vi "Process Outgoing Frames.vi"(8 "error in (no error)":errorcluster, 9 "timeout ms":i32=100, 11 "Variables":T1={"Process Ref"=refnum, "Comm Ref"=refnum, "Data Refs"={"ProtectionsAndCounters.Ref"=refnum, "Signals.Ref"=refnum, "Status.Ref"=refnum, "Overrides"=refnum, "IncomingSignals.Ref"=refnum, "CtrandProtctnVld.Ref"=refnum, "RcvTime.Ref"=refnum, "TimeDiff.Ref"=refnum, "IncomingProtCtr.Ref"=refnum}, "Settings"={"Name"="", "Priority"=0, "XNET Settings"={"Database"="", "Cluster"="", "Port"="", "Baud rate [Bd]"=0, "Termination"=0, "CAN I/O Mode"=0, "FD Baud rate [Bd]"=500000, "Priority"=100, "Use Legacy"=FALSE, "FD ISO Mode"=0}, "FPGA Session"=0, "Outgoing CAN Session"="", "Outgoing Frame Count"=0, "Outgoing Frames"=[], "Incoming CAN Session"="", "Incoming Frame Count"=0, "Incoming Frames"=[], "Incoming Values"={"Signal Values"=[], "Signal Invalid Values"=[], "ProtCtr Sig Values"=[], "Timestamps"=[], "Time Differences"=[], "IDs"=[]}}, "Stream Refs"={"Addon"="", "Port"="", "Filter Ref"=refnum, "Default Filter"={"ID Filters"=[], "Direction Filter"=enum."Tx/Rx", "Type Filter"=enum."All"}, "Port Settings"={"Mode"=0, "Baud Rate"=0, "Termination"=0, "FD ISO Mode"=0, "FD Baud Rate"=0}}} {"Stream Refs"."Port Settings"."FD ISO Mode" items=["ISO", "Non ISO", "ISO Legacy"]; "Stream Refs"."Port Settings"."Termination" items=["Off", "On"]; "Stream Refs"."Port Settings"."Mode" items=["CAN 2.0", "CAN FD", "CAN FD+BRS"]; "Settings"."XNET Settings"."FD ISO Mode" items=["ISO", "Non ISO", "ISO Legacy"]; "Settings"."XNET Settings"."CAN I/O Mode" items=["CAN 2.0", "CAN FD", "CAN FD+BRS"]; "Settings"."XNET Settings"."Termination" items=["Off", "On"]}) -> (0 "error out":errorcluster, 3 "Variables out":T1={"Process Ref"=refnum, "Comm Ref"=refnum, "Data Refs"={"ProtectionsAndCounters.Ref"=refnum, "Signals.Ref"=refnum, "Status.Ref"=refnum, "Overrides"=refnum, "IncomingSignals.Ref"=refnum, "CtrandProtctnVld.Ref"=refnum, "RcvTime.Ref"=refnum, "TimeDiff.Ref"=refnum, "IncomingProtCtr.Ref"=refnum}, "Settings"={"Name"="", "Priority"=0, "XNET Settings"={"Database"="", "Cluster"="", "Port"="", "Baud rate [Bd]"=0, "Termination"=0, "CAN I/O Mode"=0, "FD Baud rate [Bd]"=500000, "Priority"=100, "Use Legacy"=FALSE, "FD ISO Mode"=0}, "FPGA Session"=0, "Outgoing CAN Session"="", "Outgoing Frame Count"=0, "Outgoing Frames"=[], "Incoming CAN Session"="", "Incoming Frame Count"=0, "Incoming Frames"=[], "Incoming Values"={"Signal Values"=[], "Signal Invalid Values"=[], "ProtCtr Sig Values"=[], "Timestamps"=[], "Time Differences"=[], "IDs"=[]}}, "Stream Refs"={"Addon"="", "Port"="", "Filter Ref"=refnum, "Default Filter"={"ID Filters"=[], "Direction Filter"=enum."Tx/Rx", "Type Filter"=enum."All"}, "Port Settings"={"Mode"=0, "Baud Rate"=0, "Termination"=0, "FD ISO Mode"=0, "FD Baud Rate"=0}}} {"Stream Refs"."Port Settings"."FD ISO Mode" items=["ISO", "Non ISO", "ISO Legacy"]; "Stream Refs"."Port Settings"."Termination" items=["Off", "On"]; "Stream Refs"."Port Settings"."Mode" items=["CAN 2.0", "CAN FD", "CAN FD+BRS"]; "Settings"."XNET Settings"."FD ISO Mode" items=["ISO", "Non ISO", "ISO Legacy"]; "Settings"."XNET Settings"."CAN I/O Mode" items=["CAN 2.0", "CAN FD", "CAN FD+BRS"]; "Settings"."XNET Settings"."Termination" items=["Off", "On"]})   [LabVIEW 2019, in "Ghost Bus Addon Engine.lvlib"]
uses:
  Ghost Bus Addon Engine.lvlib
  Types/RT Async Engine Variables.ctl
  <vilib>/NI/NIVS Inline Async API/_VS Inline Async API/Process/Process.lvclass
  <vilib>/NI/NI VeriStand Addon Network Comm/Engine/VeriStand Comm.lvclass
  Types/RT Data References.ctl
  <vilib>/NI/NIVS Inline Async API/_Data Access Engine/Data Access Engine/Types/Write.DVR.ctl
  <vilib>/NI/NIVS Inline Async API/_Data Access Engine/Access Type Classes/Write/Write.lvclass
  <vilib>/NI/NIVS Inline Async API/_Data Access Engine/Data Access Engine/Types/Read.DVR.ctl
  <vilib>/NI/NIVS Inline Async API/_Data Access Engine/Access Type Classes/Read/Read.lvclass
  Types/RT Async Engine Settings.ctl
  Addon Shared/Types/XNET Settings.ctl
  SubModules/Frame-Protection-Support/Source/Engine/Types/RT Frame Settings.ctl
  SubModules/Frame-Protection-Support/Source/Shared/Types/Exported Frame Type.ctl
  SubModules/Frame-Protection-Support/Source/Engine/Types/RT Protection Configuration.ctl
  SubModules/Frame-Protection-Support/Source/Shared/Types/Protection Type.ctl
  SubModules/Frame-Protection-Support/Source/Shared/Types/XNET Signal Configuration.ctl
  SubModules/Frame-Protection-Support/Source/Shared/Types/Exported Counter Settings.ctl
  SubModules/Frame-Protection-Support/Source/Shared/Types/Exported Event Trigger Type.ctl
  SubModules/Frame-Protection-Support/Source/Engine/Types/RT Frame Incoming Values.ctl
  SubModules/CAN-Streaming-Support/Source/Addon/Addon Engine/Types/Engine Stream Refs.ctl
  SubModules/CAN-Streaming-Support/Source/Addon/Addon Shared/Types/Direction Filter.ctl
  SubModules/CAN-Streaming-Support/Source/Addon/Addon Shared/Types/Type Filter.ctl
  SubModules/CAN-Streaming-Support/Source/Addon/Addon Shared/Types/Filter Parameters.ctl
  SubModules/CAN-Streaming-Support/Source/Addon/Addon Engine/Types/Engine Stream Port Settings.ctl
  <vilib>/NI/NIVS Inline Async API/_Data Access Engine/Access Type Classes/Read/Read.lvclass/Read.ctl
  <vilib>/NI/NIVS Inline Async API/_Data Access Engine/Access Type Classes/Write/Write.lvclass/Write.ctl
  <vilib>/NI/NIVS Inline Async API/_Data Access Engine/Data Access Engine/Methods/Write.Data.vi
  <vilib>/NI/NIVS Inline Async API/_Data Access Engine/Access Type Classes/Write/Write.ProcessData.vi
  <vilib>/NI/NIVS Inline Async API/_Data Access Engine/Data Access Engine/Methods/Read.Data.Detect.vi
  <vilib>/NI/NIVS Inline Async API/_Data Access Engine/Data Access Engine/Methods/Read.Data.vi
  SubModules/Frame-Protection-Support/Source/Engine/SubVIs/Determine Transmit.vi
  SubModules/Frame-Protection-Support/Source/Engine/SubVIs/Update Counter Signals.vi
  SubModules/Frame-Protection-Support/Source/Engine/SubVIs/Get Frame Data.vi
  SubModules/Frame-Protection-Support/Source/Engine/SubVIs/Convert EU Data to XNET Frame.vi
  SubModules/Frame-Protection-Support/Source/Engine/SubVIs/Update Protection Signals.vi
  SubModules/Frame-Protection-Support/Source/Engine/SubVIs/Determine Disabled.vi
  <vilib>/NI/NIVS Inline Async API/_Data Access Engine/Data Access Engine/Methods/Write.Data.Commit.vi
  <vilib>/NI/NIVS Inline Async API/_Data Access Engine/Access Type Classes/Write/Write.Buffer.vi
  <vilib>/NI/NIVS Inline Async API/_Data Access Engine/Access Type Classes/Write/Write.Commit.vi
  <vilib>/NI/NIVS Inline Async API/_Data Access Engine/Access Type Classes/Read/Read.ProcessData.Detect.vi
  <vilib>/NI/NIVS Inline Async API/_Data Access Engine/Access Type Classes/Read/Read.ProcessData.vi
  SubModules/Frame-Protection-Support/Source/Engine/SubVIs/Determine Transmission.vi
  SubModules/Frame-Protection-Support/Source/Engine/SubVIs/Determine Periodic.vi
  SubModules/Frame-Protection-Support/Source/Engine/SubVIs/Set Counter Signal.vi
  SubModules/Frame-Protection-Support/Source/Engine/SubVIs/Calculate Counter Value.vi
  SubModules/Frame-Protection-Support/Source/Engine/SubVIs/Set Protection Signal.vi
  SubModules/Frame-Protection-Support/Source/Engine/SubVIs/Calculate Protection Value.vi
  <vilib>/NI/NIVS Inline Async API/_Data Access Engine/Data Access Engine/Methods/Write.Data.Buffer.vi
  SubModules/Frame-Protection-Support/Source/Engine/SubVIs/Get Protection Signals.vi
  <vilib>/xnet/xnet.llb/XNET Convert.vi
  <vilib>/xnet/xnet.llb/XNET Convert (Signal to Frame Raw).vi
  <vilib>/xnet/xnet.llb/XNET Convert (Signal to Frame CAN).vi
  <vilib>/xnet/xnet.llb/XNET Write (Frame CAN).vi
  <vilib>/NI/NIVS Inline Async API/_Data Access Engine/Data Access Engine/Data Access Engine.lvclass
  SubModules/Frame-Protection-Support/Source/Engine/Protection and Counter Support Engine.lvlib
  SubModules/Frame-Protection-Support/Source/Shared/Protection and Counter Support Shared.lvlib
  SubModules/CAN-Streaming-Support/Source/Addon/Addon Shared/CAN Stream Support Shared.lvlib
  SubModules/CAN-Streaming-Support/Source/Addon/Addon Engine/CAN Stream Support Engine.lvlib
  Addon Shared/Ghost Bus Addon Shared.lvlib
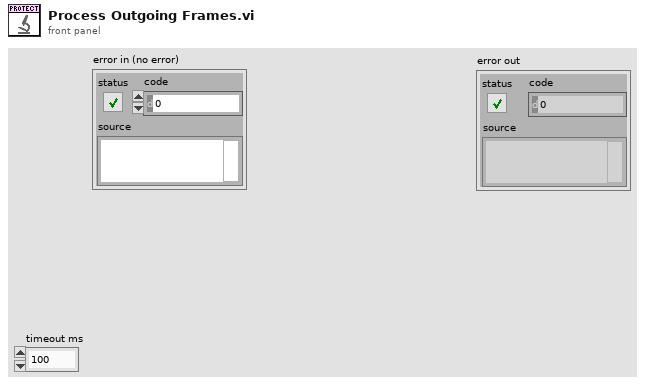
[diagram p1: front panel]
types:
  T1 = typedef "Ghost Bus Addon Engine.lvlib/RT Async Engine Variables.ctl" = cluster{"Process Ref":refnum<class "Process.lvclass">, "Comm Ref":refnum<class "VeriStand Comm.lvclass">, "Data Refs":T2, "Settings":T5, "Stream Refs":T15}
  T2 = typedef "Ghost Bus Addon Engine.lvlib/RT Data References.ctl" = cluster{"ProtectionsAndCounters.Ref":T3, "Signals.Ref":T4, "Status.Ref":T3, "Overrides":T4, "IncomingSignals.Ref":T3, "CtrandProtctnVld.Ref":T3, "RcvTime.Ref":T3, "TimeDiff.Ref":T3, "IncomingProtCtr.Ref":T3}
  T3 = typedef "Data Access Engine.lvlib/Data Access Engine.lvclass/Write.DVR.ctl" = refnum<data-value>
  T4 = typedef "Data Access Engine.lvlib/Data Access Engine.lvclass/Read.DVR.ctl" = refnum<data-value>
  T5 = typedef "Ghost Bus Addon Engine.lvlib/RT Async Engine Settings.ctl" = cluster{"Name":string, "Priority":i32, "XNET Settings":T6, "FPGA Session":u32, "Outgoing CAN Session":refnum<k21>, "Outgoing Frame Count":i32, "Outgoing Frames":T7[], "Incoming CAN Session":refnum<k21>, "Incoming Frame Count":i32, "Incoming Frames":T7[], "Incoming Values":T14}
  T6 = typedef "Ghost Bus Addon Shared.lvlib/XNET Settings.ctl" = cluster{"Database":refnum<k21>, "Cluster":refnum<k21>, "Port":string, "Baud rate [Bd]":u64, "Termination":u32, "CAN I/O Mode":u32, "FD Baud rate [Bd]":u64, "Priority":i32, "Use Legacy":bool, "FD ISO Mode":u32}
  T7 = typedef "Protection and Counter Support Engine.lvlib/RT Frame Settings.ctl" = cluster{"Type":T8, "Frame ID":u32, "Payload Length":u32, "VS Offset":i32, "VS Length":i32, "Frame Conversion":refnum<k21>, "Frame.Data":dbl[], "Generation Period":u32, "Time Since Last Generation":u32, "Generation Iterations":u32, "Generation Counter":u32, "Has Protection?":bool, "Protection Configurations":T9[], "Has Counter?":bool, "Counter Configurations":T12[], "Has Disable?":bool, "Disable VS Index":i32, "Transmit Trigger":T13, "Trigger VS Index":i32}
  T8 = typedef "Protection and Counter Support Shared.lvlib/Exported Frame Type.ctl" = enum16{"Periodic", "Event", "Periodic/Event"}
  T9 = typedef "Protection and Counter Support Engine.lvlib/RT Protection Configuration.ctl" = cluster{"Protection Frame Index":i32, "Protection Type":T10, "Data Indeces":i32[], "Data Array":dbl[], "Check Sum Conversion":refnum<k21>, "CRC Channels":T11[], "Protection VS Index":i32, "Counter Data Index":i32, "Override Index":i32, "Override Value Index":i32}
  T10 = typedef "Protection and Counter Support Shared.lvlib/Protection Type.ctl" = enum16{"Arb ID + Bytes Checksum with Inversion", "Arb ID + Bytes CRC with Inversion", "Reversed Raw Signal Checksum with Inversion", "Concatenated Two's Compliment"}
  T11 = typedef "Protection and Counter Support Shared.lvlib/XNET Signal Configuration.ctl" = cluster{"Start Bit":i32, "Name":string, "Number of bits":i32, "Scale":dbl, "Offset":dbl, "Data Type":u32, "Counter":bool}
  T12 = typedef "Protection and Counter Support Shared.lvlib/Exported Counter Settings.ctl" = cluster{"Frame Index":i32, "Max Count":dbl, "VS Index":i32, "Bit Length":i64, "Override Index":i32, "Override Value Index":i32}
  T13 = typedef "Protection and Counter Support Shared.lvlib/Exported Event Trigger Type.ctl" = enum16{"Channel value change", "Trigger channel (not zero)", "Channel value change or trigger channel (not zero)", "Trigger channel (any value change)", "Channel value change or trigger channel (any value change)"}
  T14 = typedef "Protection and Counter Support Engine.lvlib/RT Frame Incoming Values.ctl" = cluster{"Signal Values":dbl[], "Signal Invalid Values":dbl[], "ProtCtr Sig Values":dbl[], "Timestamps":timestamp[], "Time Differences":dbl[], "IDs":u32[]}
  T15 = typedef "CAN Stream Support Engine.lvlib/Engine Stream Refs.ctl" = cluster{"Addon":string, "Port":refnum<k21>, "Filter Ref":refnum<data-value>, "Default Filter":T16, "Port Settings":T19}
  T16 = typedef "CAN Stream Support Shared.lvlib/Filter Parameters.ctl" = cluster{"ID Filters":u32[], "Direction Filter":T17, "Type Filter":T18}
  T17 = typedef "CAN Stream Support Shared.lvlib/Direction Filter.ctl" = enum16{"Tx/Rx", "Rx", "Tx"}
  T18 = typedef "CAN Stream Support Shared.lvlib/Type Filter.ctl" = enum16{"All", "CAN Data", "CAN Remote", "CAN Bus Error", "CAN 2.0 Data", "CAN FD Data", "CAN FD+BRS Data", "J1939 Data", "Delay", "Log Trigger", "Start Trigger"}
  T19 = typedef "CAN Stream Support Engine.lvlib/Engine Stream Port Settings.ctl" = cluster{"Mode":u32, "Baud Rate":u64, "Termination":u32, "FD ISO Mode":u32, "FD Baud Rate":u64}
  T20 = typedef "XNET Frame CAN.ctl" = cluster{"timestamp":timestamp, "payload":u8[], "identifier":u32, "type":T21, "extended?":bool, "echo?":bool}
  T21 = typedef "XNET Frame Type CAN.ctl" = u8
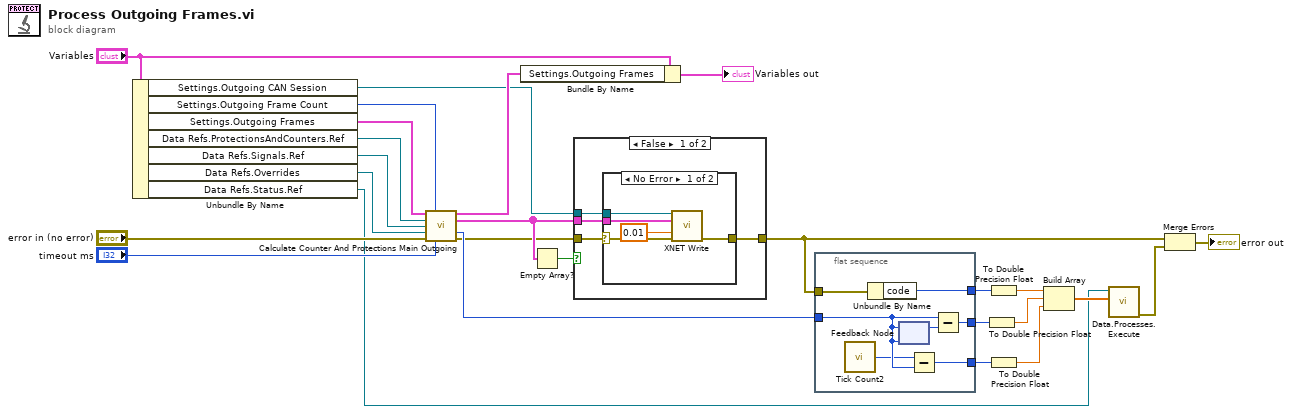
[diagram p0: block diagram]
diagram:
  n1 = Unbundle By Name("Variables") -> ("Settings.Outgoing CAN Session"=w10:refnum<k21>, "Settings.Outgoing Frame Count"=w24:i32, "Settings.Outgoing Frames"=w7:T7[], "Data Refs.ProtectionsAndCounters.Ref"=w2:T3, "Data Refs.Signals.Ref"=w3:T4, "Data Refs.Overrides"=w1:T4, "Data Refs.Status.Ref"=w4:T3)
  n2 = call "Calculate Counter And Protections Main Outgoing.vi"("Frames in"=w7, "Frame Count"=w24, "Protections"=w2, "Signals"=w3, "Overrides"=w1, "error in (no error)"="error in (no error)", "timeout ms"="timeout ms") -> ("Frames out"=w14:T7[], "Frames"=w13:T20[], "Tick Count(uSec)"=w22:u32, "error out"=w9:errorcluster)  [unwired: 5 in]
  n3 = Bundle By Name(cluster="Variables", "Settings.Outgoing Frames"=w14) -> (→"Variables out":T1)
  n4 = Empty Array?(array=w13) -> (empty?=w12:bool)
  n5 = case shown="False" w12 {
    tunnel: w9 -> [w30 w37]
    tunnel: [w29 w37] -> w8
    tunnel: w10 -> [w28 _]
    tunnel: w13 -> [w27 _]
    frame False {
      n6 = case shown="No Error" w30 {
        selector: w30 -> [w32 w36]
        tunnel: w27 -> [w35 _]
        tunnel: [w34 w36] -> w29
        tunnel: w28 -> [w33 _]
        frame No Error {
          n7 = call-poly <vilib>:"XNET Write.vi"("session in"=w33, "data"=w35, "timeout (10)"=0.01, "error in (no error)"=w32) -> ("error out"=w34:errorcluster)  [unwired: 10 in, 1 out]
        }
        frame Error {
        }
      }
    }
    frame True {
    }
  }
  n8 = flat-sequence {
    tunnel: w22 -> [w44]
    tunnel: [w43] -> w21
    tunnel: [w42] -> w18
    tunnel: w8 -> [w39]
    tunnel: [w38] -> w11
    frame #0 {
      n9 = call "Tick Count2"() -> ("Tick Count(uSec)"=w41:u32)
      n10 = Unbundle By Name(w39) -> ("code"=w38:i32)
      n11 = feedback #1(w44) -> (w40:u32)
      n12 = feedback-in #1(w44) -> ()
      n13 = Subtract(x=w41, y=w44) -> (x-y=w42:u32)
      n14 = Subtract(x=w44, y=w40) -> (x-y=w43:u32)
    }
  }
  n15 = To Double Precision Float(number=w21) -> (double precision float=w16:dbl)
  n16 = To Double Precision Float(number=w11) -> (double precision float=w17:dbl)
  n17 = To Double Precision Float(number=w18) -> (double precision float=w15:dbl)
  n18 = Build Array(w17, w16, w15) -> (w20:dbl[])
  n19 = call-poly <vilib>:"Data.Processes.Execute.vi"("Values"=w20, "Ref"=w4) -> ("error out"=w19:errorcluster)  [unwired: 9 in]
  n20 = Merge Errors(w8, w19) -> (→"error out":errorcluster)
